vi "FTC Read Packet Flush.vi"(3 "Mailbox":T1 items=["Mailbox 1", "Mailbox 2", "Mailbox 3", "Mailbox 4", "Mailbox 5", "Mailbox 6", "Mailbox 7", "Mailbox 8", "Mailbox 9", "Mailbox 10"], 5 "NXT":T2={"Hardware"="NXT", "Flattened String"=""}) -> (0 "Message":string, 1 "Packet Received?":bool, 2 "NXT":T2={"Hardware"="NXT", "Flattened String"=""})   [LabVIEW 2011]
doc: "Reads data that the FIRST Tech Challenge (FTC) Controller Station or field management system (FMS) sends to the NXT device. Wire the <B>Controller 1</B> or <B>Controller 2</B> output of this VI to the <B>Packet</B> input of the FTC Read Controller VI to read the data for a specific game controller.\n\nBluetooth packes are flushed from the buffer prior to each read to ensure that there is the shortest possible control lag."
uses:
  <vilib>/NXT/Subs/LVHSConnector.ctl
  <vilib>/NXT/Block Support/NXT_MessageMailbox.ctl
  <vilib>/NXT/Dual Mode Library/BT/BlueTooth_Read_string.vi
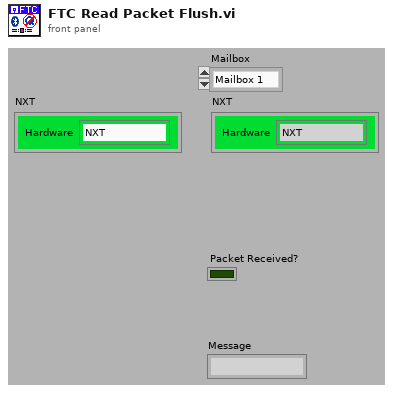
[diagram p1: front panel]
types:
  T1 = typedef "NXT_MessageMailbox.ctl" = u8
  T2 = typedef "LVHSConnector.ctl" = cluster{"Hardware":string, "Flattened String":string}
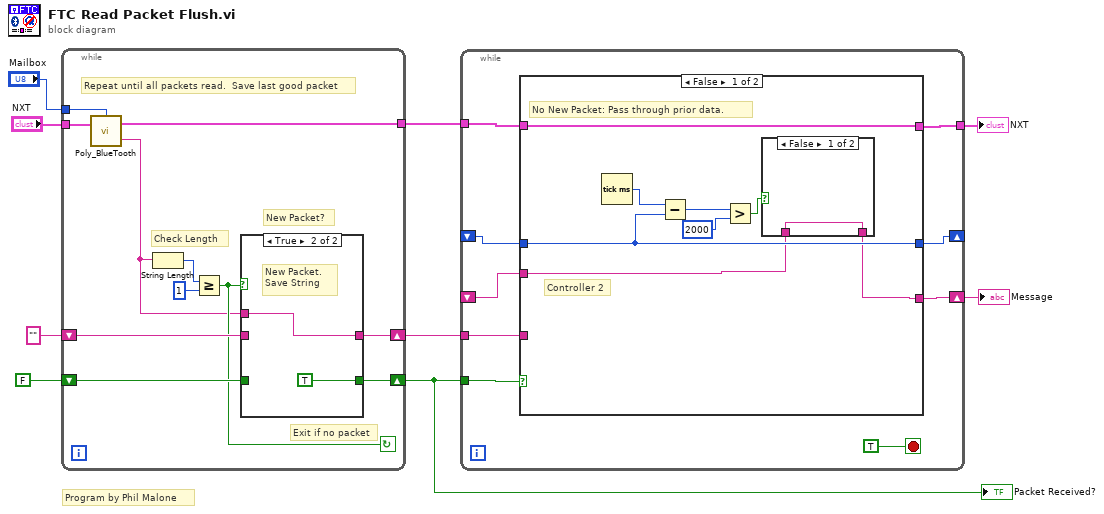
[diagram p0: block diagram]
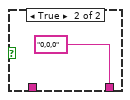
[diagram p2: hidden frame]
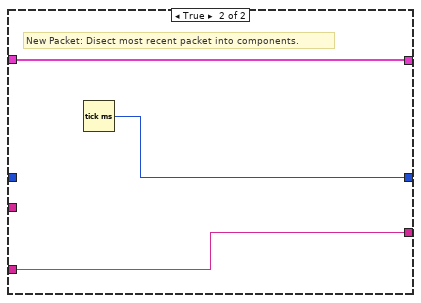
[diagram p3: hidden frame]
diagram:
  # "Program by Phil Malone"
  n1 = while {
    tunnel: "NXT" -> [w20]
    tunnel: [w19] -> w6
    shift-right: [w16] -> w5
    shift-left: "" ("Message") -> [w15]
    shift-right: [w14] -> w2
    shift-left: FALSE -> [w13]
    tunnel: "Mailbox" -> [w10]
    stop <- w12 continue-if-true
    # "Exit if no packet"
    # "Check Length"
    # "Repeat until all packets read.  Save last good packet"
    # "New Packet?"
    n2 = call-poly <vilib>:"Poly_BlueTooth.vi"("NXT"=w20, "Mailbox"=w10) -> ("Message"=w11:string, "NXT"=w19:T2)  [unwired: 1 in]
    n3 = String Length(string=w11) -> (length=w17:i32)
    n4 = Greater Or Equal?(x=w17, y=1 ("Packet Length")) -> (x >= y?=w12:bool)
    n5 = case shown="True" w12 {
      tunnel: w11 -> [_ w24]
      tunnel: [w22 w24] -> w16
      tunnel: w15 -> [w22 _]
      tunnel: [w21 TRUE] -> w14
      tunnel: w13 -> [w21 _]
      frame False {
        # "No Packet.  \nDo Nothing"
      }
      frame True {
        # "New Packet.  \nSave String"
      }
    }
  }
  "Packet Received?" <- w2
  n6 = while {
    tunnel: [w32] -> w8
    tunnel: w6 -> [w31]
    tunnel: w5 -> [w30]
    tunnel: w2 -> [w29]
    shift-right: [w33] -> w9
    shift-left: _ -> [w27]
    shift-right: [w26] -> _
    shift-left: _ -> [w25]
    stop <- TRUE stop-if-true
    n7 = case shown="False" w29 {
      tunnel: [w34 w45] -> w33
      tunnel: w30 -> [_ w45]
      tunnel: w31 -> [w41 w46]
      tunnel: [w41 w46] -> w32
      tunnel: w27 -> [w36 _]
      tunnel: [w39 w44] -> w26
      tunnel: w25 -> [w39 _]
      frame False {
        # "Controller 2"
        # "No New Packet: Pass through prior data."
        n8 = Tick Count (ms)() -> (millisecond timer value=w40:u32)
        n9 = Subtract(x=w40, y=w39) -> (x-y=w38:u32)
        n10 = Greater?(x=w38, y=u32 2000) -> (0:w35:bool)
        n11 = case shown="False" w35 {
          tunnel: w36 -> [w42 _]
          tunnel: [w42 "0,0,0"] -> w34
          frame False {
          }
          frame True {
          }
        }
      }
      frame True {
        # "New Packet: Disect most recent packet into components."
        n12 = Tick Count (ms)() -> (millisecond timer value=w44:u32)
      }
    }
  }
  "Message" <- w9
  "NXT" <- w8
